vi "Group 1-Char Tokens.vi"(10 "Raw Tokens":string[](array[string])) -> (2 "Grouped Tokens":string[](array[string]))   [LabVIEW 2014]
doc: "Copyright (c) 2020 Sze Howe Koh\n\nThis Source Code Form is subject to the terms of the Mozilla Public License, v. 2.0. If a copy of the MPL was not distributed with this file, You can obtain one at http://mozilla.org/MPL/2.0/."
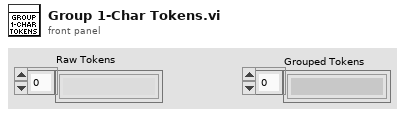
[diagram p1: front panel]
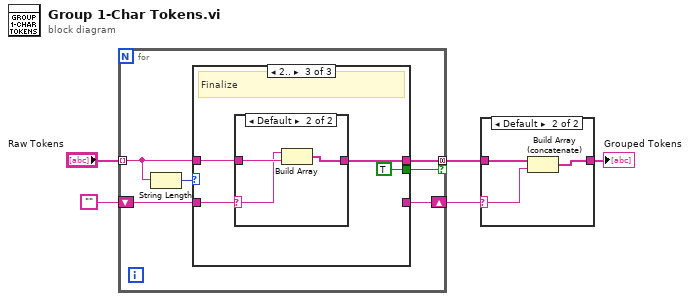
[diagram p0: block diagram]
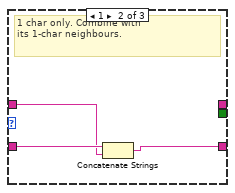
[diagram p4: hidden frame]
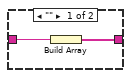
[diagram p5: hidden frame]
diagram:
  n1 = for {
    tunnel: "Raw Tokens" -> [w7] mode=indexing
    shift-right: [w9] -> w2
    shift-left: "" -> [w8]
    tunnel: [w6] -> w3 mode=concatenating if=w10
    n2 = String Length(string=w7) -> (length=w11:i32)
    n3 = case shown="2.." w11 {
      tunnel: w7 -> [_ w14 w18]
      tunnel: [_ _ w17] -> w6
      tunnel: [_ _ TRUE] -> w10
      tunnel: [w12 w13 _] -> w9
      tunnel: w8 -> [w12 w15 w16]
      frame ..0 {
        # "Shouldn't happen"
      }
      frame 1 {
        # "1 char only. Combine with\nits 1-char neighbours."
        n4 = Concatenate Strings(w15, w14) -> (w13:string)
      }
      frame 2.. {
        # "Finalize"
        n5 = case shown="Default" w16 {
          selector: w16 -> [_ w22]
          tunnel: w18 -> [w21 w24]
          tunnel: [w20 w23] -> w17
          frame "" {
            n6 = Build Array(w21) -> (w20:string[])
          }
          frame Default {
            n7 = Build Array(w22, w24) -> (w23:string[])
          }
        }
      }
    }
  }
  n8 = case shown="Default" w2 {
    selector: w2 -> [_ w26]
    tunnel: w3 -> [w25 w28]
    tunnel: [w25 w27] -> w1
    frame "" {
    }
    frame Default {
      n9 = Build Array (concatenate)(w28, w26) -> (w27:string[])
    }
  }
  "Grouped Tokens" <- w1
